vi "GetMetricTagId.vi"(8 "error in (no error)":errorcluster, 10 "tags":T1[](array[typedef]), 11 "metric id":string) -> (0 "error out":errorcluster, 1 "tag id":string, 3 "found":bool)   [LabVIEW 2017, in "DeviceModelHelpers.lvlib"]
doc: "Returns the corresponding tag ID for the specified metric ID."
uses:
  <vilib>/addons/InsightCM/Utilities/DeviceModelHelpers/DeviceModelHelpers.lvlib
  <vilib>/addons/InsightCM/MessageBus/Base/controls/Tag.ctl
  <vilib>/addons/InsightCM/MessageBus/Base/controls/KeyValuePair.ctl
  <vilib>/addons/InsightCM/Utilities/PropertyHelpers/PropertyHelpers.lvlib
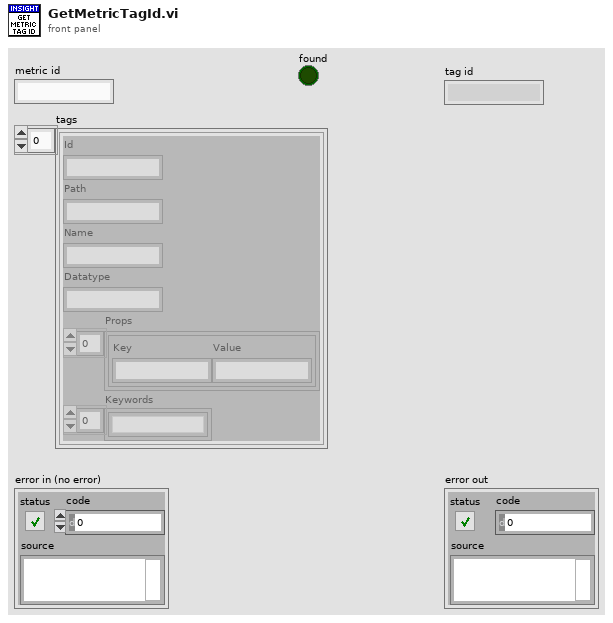
[diagram p1: front panel]
types:
  T1 = typedef "Tag.ctl" = cluster{"Id":string, "Path":string, "Name":string, "Datatype":string, "Props":T2[], "Keywords":string[]}
  T2 = typedef "KeyValuePair.ctl" = cluster{"Key":string, "Value":string}
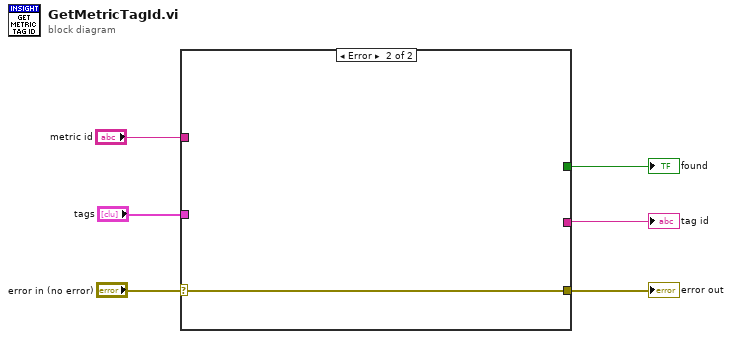
[diagram p0: block diagram]
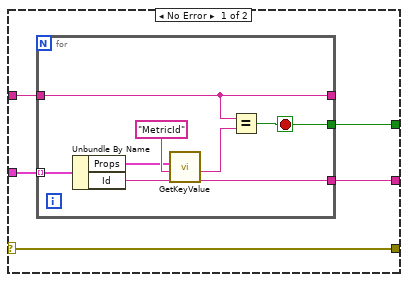
[diagram p2: hidden frame]
diagram:
  n1 = case shown="Error" "error in (no error)" {
    selector: "error in (no error)" -> [w8 w19]
    tunnel: "metric id" -> [w11 _]
    tunnel: "tags" -> [w10 _]
    tunnel: [w9 _] -> w2
    tunnel: [w8 w19] -> w3
    tunnel: [w7 _] -> w1
    frame No Error {
      n2 = for {
        tunnel: w11 -> [w15]
        tunnel: w10 -> [w18] mode=indexing
        tunnel: [w17] -> w9
        tunnel: [w16] -> w7
        tunnel: [w15] -> _
        stop <- w16 stop-if-true
        n3 = Unbundle By Name(w18) -> ("Props"=w12:T2[], "Id"=w17:string)
        n4 = call <vilib>:"GetKeyValue.vi"("key"="MetricId", "key value pairs"=w12) -> ("value"=w14:string)  [unwired: 7 in, 2 out]
        n5 = Equal?(x=w15, y=w14) -> (x = y?=w16:bool)
      }
    }
    frame Error {
    }
  }
  "error out" <- w3
  "tag id" <- w2
  "found" <- w1
